vi "Read Data From '.id' Files1.vi"(1 "ID File Path":string="\\\\beco\\autoage\\id\\", 3 "ID Filename":string) -> (0 "# Days for Aging Spec":string, 2 "PISN #":string, 4 "Gate Time":string, 5 "Aging Spec":string, 6 "Unit Type":string, 7 "Customer":string, 8 "Nominal Frequency":string, 9 "Aging Spec 2":string)   [LabVIEW 2021]
panel:
  # "MHz"
  # "sec"
  # "ppm"
  # "ppb/day"
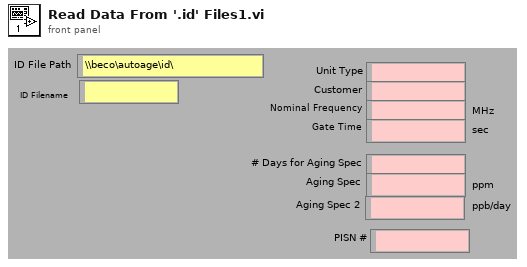
[diagram p1: front panel]
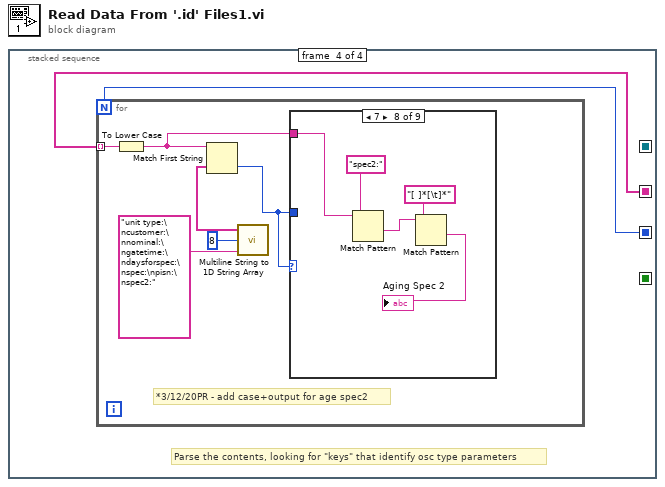
[diagram p0: block diagram]
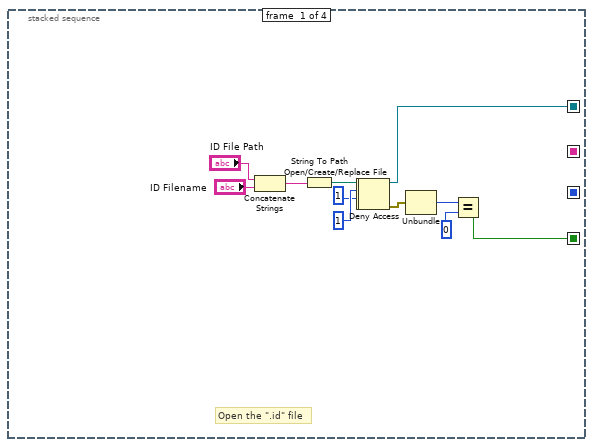
[diagram p2: hidden frame]
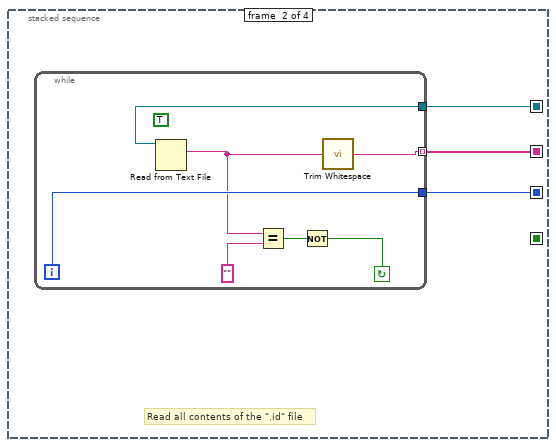
[diagram p3: hidden frame]
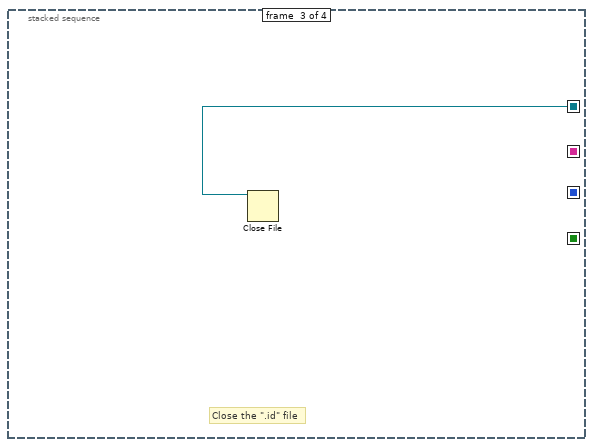
[diagram p4: hidden frame]
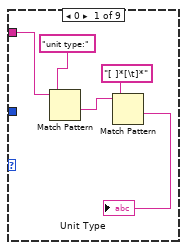
[diagram p5: hidden frame]
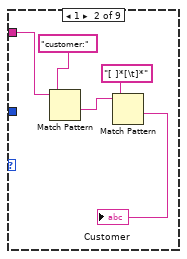
[diagram p6: hidden frame]
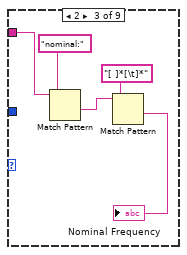
[diagram p7: hidden frame]
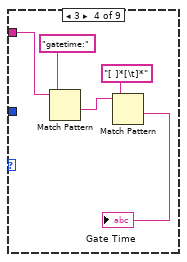
[diagram p8: hidden frame]
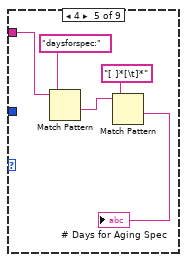
[diagram p9: hidden frame]
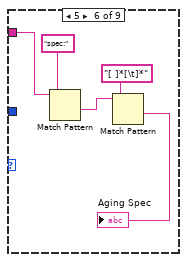
[diagram p10: hidden frame]
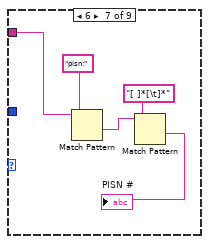
[diagram p11: hidden frame]
diagram:
  n1 = stacked-sequence {
    seq-local: [w6 _ _ _] -> [_ w16 w24 _]
    seq-local: [w5 _ _ _] -> [_ _ _ _]
    seq-local: [_ w15 _ _] -> [_ _ _ w26]
    seq-local: [_ w14 _ _] -> [_ _ _ w25]
    frame #0 {
      # "Open the \".id\" file"
      n2 = Concatenate Strings("ID File Path", "ID Filename") -> (w13:string)
      n3 = String To Path(string=w13) -> (path=w12:path)
      n4 = Open/Create/Replace File(file path (use dialog)=w12, access (0:read/write)=1) -> (refnum out=w1:refnum<file>, error out=w2:errorcluster)  [unwired: 4 in, 1 out]
      n5 = Deny Access(4:w2, 6:1, 7:w1) -> (0:w9:errorcluster, 3:w6:refnum<file>)
      n6 = Unbundle(w9) -> ("code"=w7:i32)  [unwired: 2 out]
      n7 = Equal?(x=w7, y=0) -> (x = y?=w5:bool)
    }
    frame #1 {
      # "Read all contents of the \".id\" file"
      n8 = while {
        tunnel: [w19] -> w14
        tunnel: [w17] -> w15 mode=indexing
        tunnel: w16 -> [w20]
        i -> [w19]
        stop <- w21 continue-if-true
        (unwired) TRUE
        n9 = Read from Text File(file (use dialog)=w20) -> (text=w18:string)  [unwired: 3 in, 3 out]
        n10 = Equal?(x=w18, y="") -> (x = y?=w22:bool)
        n11 = Not(x=w22) -> (.not. x?=w21:bool)
        n12 = call <vilib>:"Trim Whitespace.vi"("string"=w18) -> ("trimmed string"=w17:string)  [unwired: 1 in]
      }
    }
    frame #2 {
      # "Close the \".id\" file"
      n13 = Close File(refnum=w24) -> ()  [unwired: 1 in, 2 out]
    }
    frame #3 {
      # "Parse the contents, looking for \"keys\" that identify osc type parameters"
      n14 = for {
        N: w25 -> [_]
        tunnel: w26 -> [w30] mode=indexing
        # "*3/12/20PR - add case+output for age spec2"
        n15 = To Lower Case(string=w30) -> (all lower case string=w27:string)
        n16 = call "Multiline String to 1D String Array.vi"("Multiline Input String"="unit type:\ncustomer:\nnominal:\ngatetime:\ndaysforspec:\nspec:\npisn:\nspec2:", "Number of Elements"=8) -> ("1D String Output Array"=w29:string[])
        n17 = Match First String(2:w29, 3:w27) -> (0:w28:i32)  [unwired: 1 out]
        n18 = case shown="7" w28 {
          tunnel: w27 -> [w37 w42 w47 w52 w57 w62 w64 w69 _]
          tunnel: w28 -> [_ _ _ _ _ _ _ _ _]
          frame 0 {
            n19 = Match Pattern(string=w37, regular expression="unit type:") -> (after substring=w34:string)  [unwired: 1 in, 3 out]
            n20 = Match Pattern(string=w34, regular expression="[ ]*[\t]*") -> (after substring=→"Unit Type":string)  [unwired: 1 in, 3 out]
          }
          frame 1 {
            n21 = Match Pattern(string=w42, regular expression="customer:") -> (after substring=w39:string)  [unwired: 1 in, 3 out]
            n22 = Match Pattern(string=w39, regular expression="[ ]*[\t]*") -> (after substring=→"Customer":string)  [unwired: 1 in, 3 out]
          }
          frame 2 {
            n23 = Match Pattern(string=w47, regular expression="nominal:") -> (after substring=w44:string)  [unwired: 1 in, 3 out]
            n24 = Match Pattern(string=w44, regular expression="[ ]*[\t]*") -> (after substring=→"Nominal Frequency":string)  [unwired: 1 in, 3 out]
          }
          frame 3 {
            n25 = Match Pattern(string=w52, regular expression="gatetime:") -> (after substring=w49:string)  [unwired: 1 in, 3 out]
            n26 = Match Pattern(string=w49, regular expression="[ ]*[\t]*") -> (after substring=→"Gate Time":string)  [unwired: 1 in, 3 out]
          }
          frame 4 {
            n27 = Match Pattern(string=w57, regular expression="daysforspec:") -> (after substring=w54:string)  [unwired: 1 in, 3 out]
            n28 = Match Pattern(string=w54, regular expression="[ ]*[\t]*") -> (after substring=→"# Days for Aging Spec":string)  [unwired: 1 in, 3 out]
          }
          frame 5 {
            n29 = Match Pattern(string=w62, regular expression="spec:") -> (after substring=w59:string)  [unwired: 1 in, 3 out]
            n30 = Match Pattern(string=w59, regular expression="[ ]*[\t]*") -> (after substring=→"Aging Spec":string)  [unwired: 1 in, 3 out]
          }
          frame 6 {
            n31 = Match Pattern(string=w64, regular expression="pisn:") -> (after substring=w65:string)  [unwired: 1 in, 3 out]
            n32 = Match Pattern(string=w65, regular expression="[ ]*[\t]*") -> (after substring=→"PISN #":string)  [unwired: 1 in, 3 out]
          }
          frame 7 {
            n33 = Match Pattern(string=w69, regular expression="spec2:") -> (after substring=w70:string)  [unwired: 1 in, 3 out]
            n34 = Match Pattern(string=w70, regular expression="[ ]*[\t]*") -> (after substring=→"Aging Spec 2":string)  [unwired: 1 in, 3 out]
          }
          frame -1, Default {
          }
        }
      }
    }
  }
